vi "Preview Sample.vi"(8 "error in (no error)":errorcluster, 9 "Queue timeout in ms (-1)":i32=-1, 11 "He Line in":refnum<class "He Line.lvclass">) -> (0 "error out":errorcluster, 1 "Queue timed out?":bool, 2 "element":refnum<class "Sample.lvclass">, 3 "He Line out":refnum<class "He Line.lvclass">)   [LabVIEW 2015, in "cRIO-Carbondioxide.lvlib" / "CO2-Actor.lvlib" / "He Line.lvclass"]
uses:
  He Line.lvclass
  subs/Sample/Sample.lvclass
  He Line.lvclass/He Line.ctl
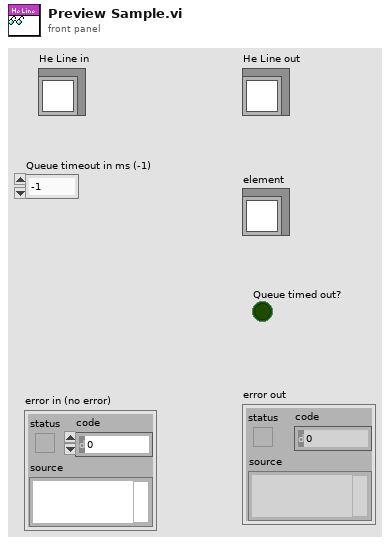
[diagram p1: front panel]
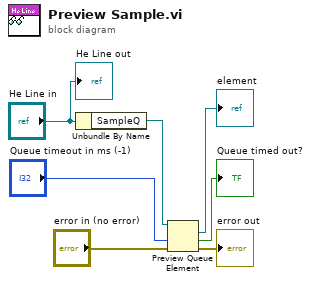
[diagram p0: block diagram]
diagram:
  n1 = Unbundle By Name("He Line in") -> ("SampleQ"=w5:refnum<queue>)
  n2 = Preview Queue Element(queue=w5, timeout in ms (-1)="Queue timeout in ms (-1)", error in (no error)="error in (no error)") -> (element=→"element":refnum<class "Sample.lvclass">, timed out?=→"Queue timed out?":bool, error out=→"error out":errorcluster)  [unwired: 1 out]
  "He Line out" <- "He Line in"
